vi "Get Global VI Data.vi"(8 "error in (no error)":errorcluster, 11 "VI in":refnum<vi>) -> (0 "error out":errorcluster, 2 "VI Properties":T1, 3 "VI out":refnum<vi>)   [LabVIEW 2023, in "VI Properties Editor.lvlib"]
doc: "Gets all data for a global VI."
uses:
  VI Properties Editor.lvlib
  CTLs/VI Properties.ctl
  <vilib>/picture/picture.llb/imagedata.ctl
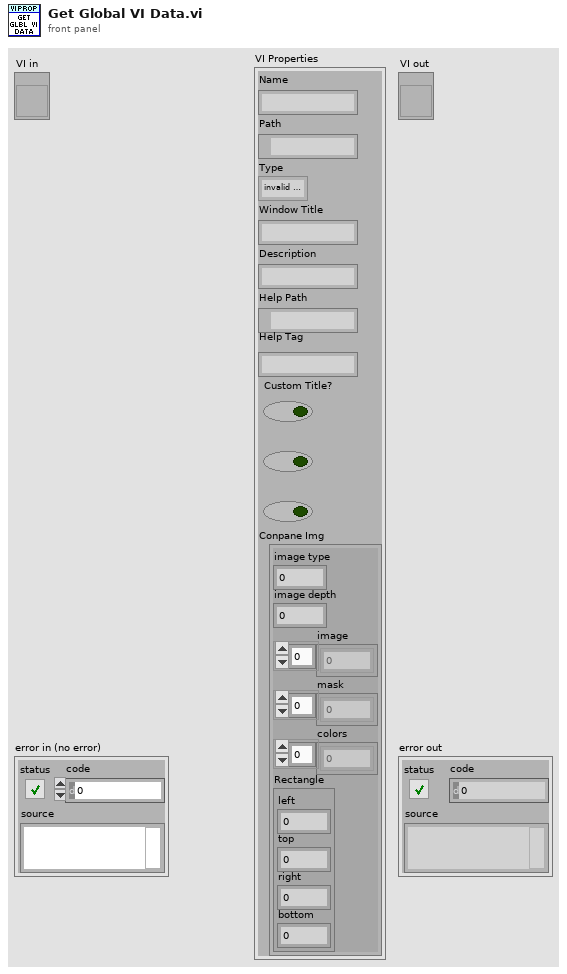
[diagram p1: front panel]
types:
  T1 = typedef "VI Properties Editor.lvlib/VI Properties.ctl" = cluster{"Name":string, "Path":path, "Type":enum32{"invalid VI type", "Standard VI", "Control VI", "Global VI", "Polymorphic VI", "Configuration VI", "SubSystem", "Facade VI", "Method VI", "Statechart Diagram VI"}, "Window Title":string, "Description":string, "Help Path":path, "Help Tag":string, "Custom Title?":bool, "Reentrant?":bool, "Inlined?":bool, "Conpane Img":T2}
  T2 = typedef "imagedata.ctl" = cluster{"image type":i32, "image depth":i32, "image":u8[], "mask":u8[], "colors":u32[], "Rectangle":cluster{"left":i16, "top":i16, "right":i16, "bottom":i16}}
  T3 = enum32{"invalid VI type", "Standard VI", "Control VI", "Global VI", "Polymorphic VI", "Configuration VI", "SubSystem", "Facade VI", "Method VI", "Statechart Diagram VI"}
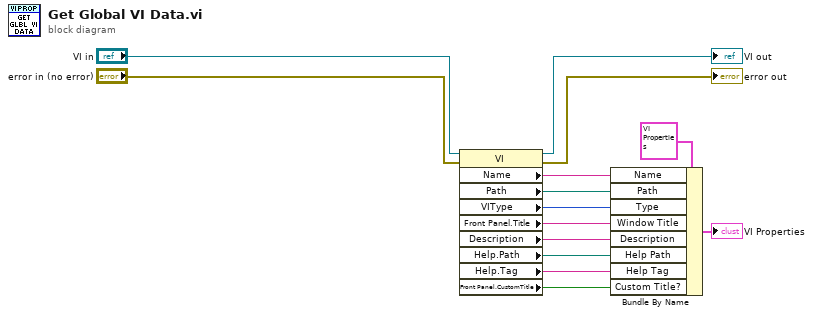
[diagram p0: block diagram]
diagram:
  n1 = property class="VI"(reference="VI in", error in="error in (no error)") -> (reference out=→"VI out":refnum<vi>, error out=→"error out":errorcluster, "Name"=w13:string, "Path"=w12:path, "VIType"=w11:T3, "Front Panel.Title"=w2:string, "Description"=w10:string, "Help.Path"=w9:path, "Help.Tag"=w8:string, "Front Panel.CustomTitle"=w1:bool)
  n2 = Bundle By Name(cluster=T1 {"Name"="", "Path"=path "", "Type"=enum."invalid VI type", "Window Title"="", "Description"="", "Help Path"=path "", "Help Tag"="", "Custom Title?"=FALSE, "Reentrant?"=FALSE, "Inlined?"=FALSE, "Conpane Img"={"image type"=0, "image depth"=0, "image"=[], "mask"=[], "colors"=[], "Rectangle"={"left"=0, "top"=0, "right"=0, "bottom"=0}}} ("VI Properties"), "Name"=w13, "Path"=w12, "Type"=w11, "Window Title"=w2, "Description"=w10, "Help Path"=w9, "Help Tag"=w8, "Custom Title?"=w1) -> (→"VI Properties":T1)
